vi "simSync_Create.vi"(8 "error in (no error)":errorcluster, 11 "reference in":refnum<class "simSync.lvclass">) -> (0 "error out":errorcluster, 3 "reference out":refnum<class "simSync.lvclass">)   [LabVIEW 2019, in "simSync.lvclass"]
doc: "Constructor."
uses:
  simSync.lvclass
  C:/Program Files/National Instruments/LabVIEW 2019/vi.lib/addons/_AddQ/G#Object/G#Object.lvclass
  C:/Barkhausen mmWave radar/Development/LV/Barkhausen mmWave hardware control/Host/SubVIs/Timing_class/Timing.lvclass
  <vilib>/addons/_AddQ/G#Object/G#Object.lvclass
  Timing_class/Timing.lvclass
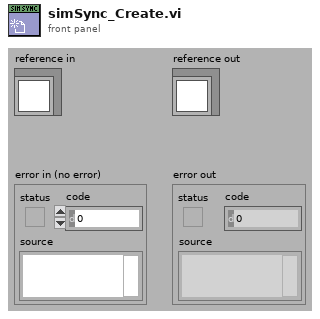
[diagram p1: front panel]
types:
  T1 = typedef "simSync.lvclass/ObjectAttributesRef.ctl" = refnum<data-value>
  T2 = typedef "simSync.lvclass/ObjectAttributes.ctl" = cluster{"MyAttribute":dbl}
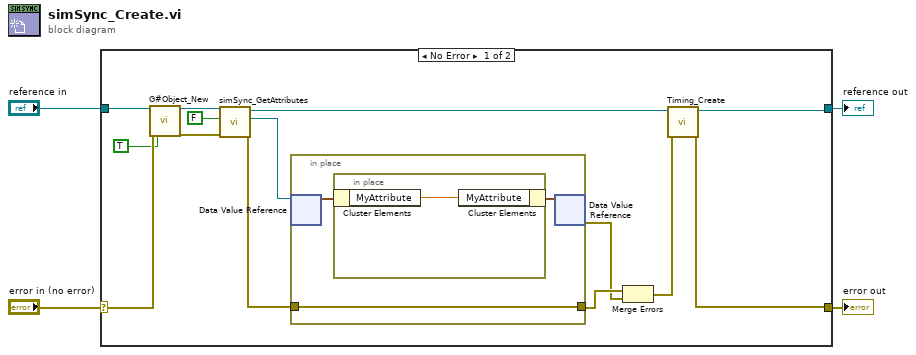
[diagram p0: block diagram]
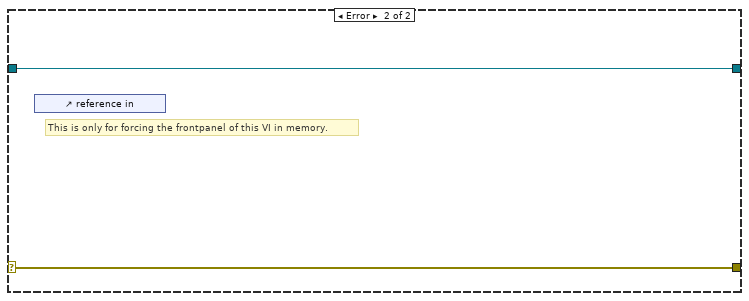
[diagram p2: hidden frame]
diagram:
  n1 = case shown="No Error" "error in (no error)" {
    selector: "error in (no error)" -> [w17 w24]
    tunnel: [w5 w24] -> w3
    tunnel: [w7 w23] -> w1
    tunnel: "reference in" -> [w18 w23]
    frame No Error {
      n2 = call <vilib>:"G#Object_New.vi"("reference in"=w18, "error in (no error)"=w17, "user counter (T)?"=TRUE ("User Counter")) -> ("reference out"=w10:refnum<class "simSync.lvclass">, "error out"=w9:errorcluster)  [unwired: 14 in, 1 out]
      n3 = call "simSync_GetAttributes.vi"("error in (no error)"=w9, "return data? (T)"=FALSE ("return data"), "reference in"=w10) -> ("error out"=w13:errorcluster, "attributes ref"=w12:T1, "reference out"=w8:refnum<class "simSync.lvclass">)  [unwired: 5 in, 1 out]
      n4 = in-place {
        in-place-border: w13 -> [w19]
        in-place-border: [w19] -> w15
        n5 = in-place-dvr #1(w12) -> (w20:T2)  [unwired: 1 out]
        n6 = in-place {
          n7 = in-place-cluster #2(w20) -> ("MyAttribute"=w22:dbl)
          n8 = in-place-cluster #2("MyAttribute"=w22) -> (w21:T2)
        }
        n9 = in-place-dvr #1(w21) -> (w14:errorcluster)  [unwired: 1 out]
      }
      n10 = Merge Errors(w15, w14) -> (w6:errorcluster)
      n11 = call "Timing_Create.vi"("error in (no error)"=w6, "reference in"=w8) -> ("error out"=w5:errorcluster, "reference out"=w7:refnum<class "simSync.lvclass">)  [unwired: 8 in]
    }
    frame Error {
      # "This is only for forcing the frontpanel of this VI in memory."
      n12 = control-ref of="reference in"() -> ()  [unwired: 1 out]
    }
  }
  "error out" <- w3
  "reference out" <- w1
